vi "CompVisionUtil_ObjectToRobotPose.vi"(9 "RobotToCamera":T1={"TRANSLATION3D"={"X"=0.0, "Y"=0.0, "Z"=0.0}, "ROTATION3D"={"Q_quaternion"={"R"=1.0, "V"=[0.0, 0.0, 0.0]}}, "XF"=FALSE} {"TRANSLATION3D"."Z" format="%14.3f"; "TRANSLATION3D"."Y" format="%14.3f"; "TRANSLATION3D"."X" format="%14.3f"}, 10 "CameraToObject":T1={"TRANSLATION3D"={"X"=0.0, "Y"=0.0, "Z"=0.0}, "ROTATION3D"={"Q_quaternion"={"R"=1.0, "V"=[0.0, 0.0, 0.0]}}, "XF"=FALSE} {"TRANSLATION3D"."Z" format="%14.3f"; "TRANSLATION3D"."Y" format="%14.3f"; "TRANSLATION3D"."X" format="%14.3f"}, 11 "ObjectInField":T5={"Translation3d"={"X"=0.0, "Y"=0.0, "Z"=0.0}, "Rotation3d"={"Q_quaternion"={"R"=1.0, "V"=[0.0, 0.0, 0.0]}}} {"Translation3d"."Z" format="%14.3f"; "Translation3d"."Y" format="%14.3f"; "Translation3d"."X" format="%14.3f"}) -> (3 "ObjectToRobotPose":T5={"Translation3d"={"X"=0.0, "Y"=0.0, "Z"=0.0}, "Rotation3d"={"Q_quaternion"={"R"=1.0, "V"=[0.0, 0.0, 0.0]}}} {"Translation3d"."Z" format="%14.3f"; "Translation3d"."Y" format="%14.3f"; "Translation3d"."X" format="%14.3f"})   [LabVIEW 2019, in "Trajectory_Library.lvlib"]
doc: "Returns the robot's pose in the field coordinate system given an object's field-relative pose, the transformation from the camera's pose to the object's pose (obtained via computer vision), and the transformation from the robot's pose to the camera's pose.\n\nThe object could be a target or a fiducial marker.\n \nInputs:\n -- ObjectInField -- Pose3d -- An object's field-relative pose.\n -- CameraToObject -- Transform3d -- The transformation from the camera's pose to the object's pose. This comes from computer vision.\n -- RobotToCamera -- Transform3d -- The transformation from the robot's pose to the camera's pose. This can either be a constant for a rigidly mounted camera, or variable if the camera is mounted to\n a turret. If the camera was mounted 3 inches in front of the \"origin\" (usually physical center) of the robot, this would be new Transform3d(Units.inchesToMeters(3.0), 0.0, 0.0,\n new Rotation3d()).\n\nReturns:\n -- ObjectToRobotPose -- Pose3d -- The robot's field-relative pose."
uses:
  Trajectory_Library.lvlib
  TypeDef/TRANSLATION3D.ctl
  TypeDef/QUATERNION.ctl
  TypeDef/ROTATION3D.ctl
  TypeDef/POSE3D.ctl
  TypeDef/TRANSFORM3D.ctl
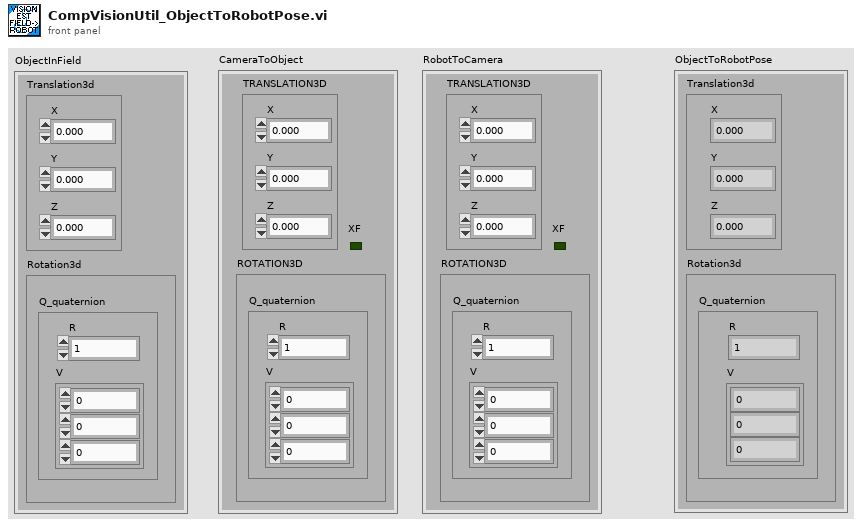
[diagram p1: front panel]
types:
  T1 = typedef "Trajectory_Library.lvlib/TRANSFORM3D.ctl" = cluster{"TRANSLATION3D":T2, "ROTATION3D":T3, "XF":bool}
  T2 = typedef "Trajectory_Library.lvlib/TRANSLATION3D.ctl" = cluster{"X":dbl, "Y":dbl, "Z":dbl}
  T3 = typedef "Trajectory_Library.lvlib/ROTATION3D.ctl" = cluster{"Q_quaternion":T4}
  T4 = typedef "Trajectory_Library.lvlib/QUATERNION.ctl" = cluster{"R":dbl, "V":dbl[]}
  T5 = typedef "Trajectory_Library.lvlib/POSE3D.ctl" = cluster{"Translation3d":T2, "Rotation3d":T3}
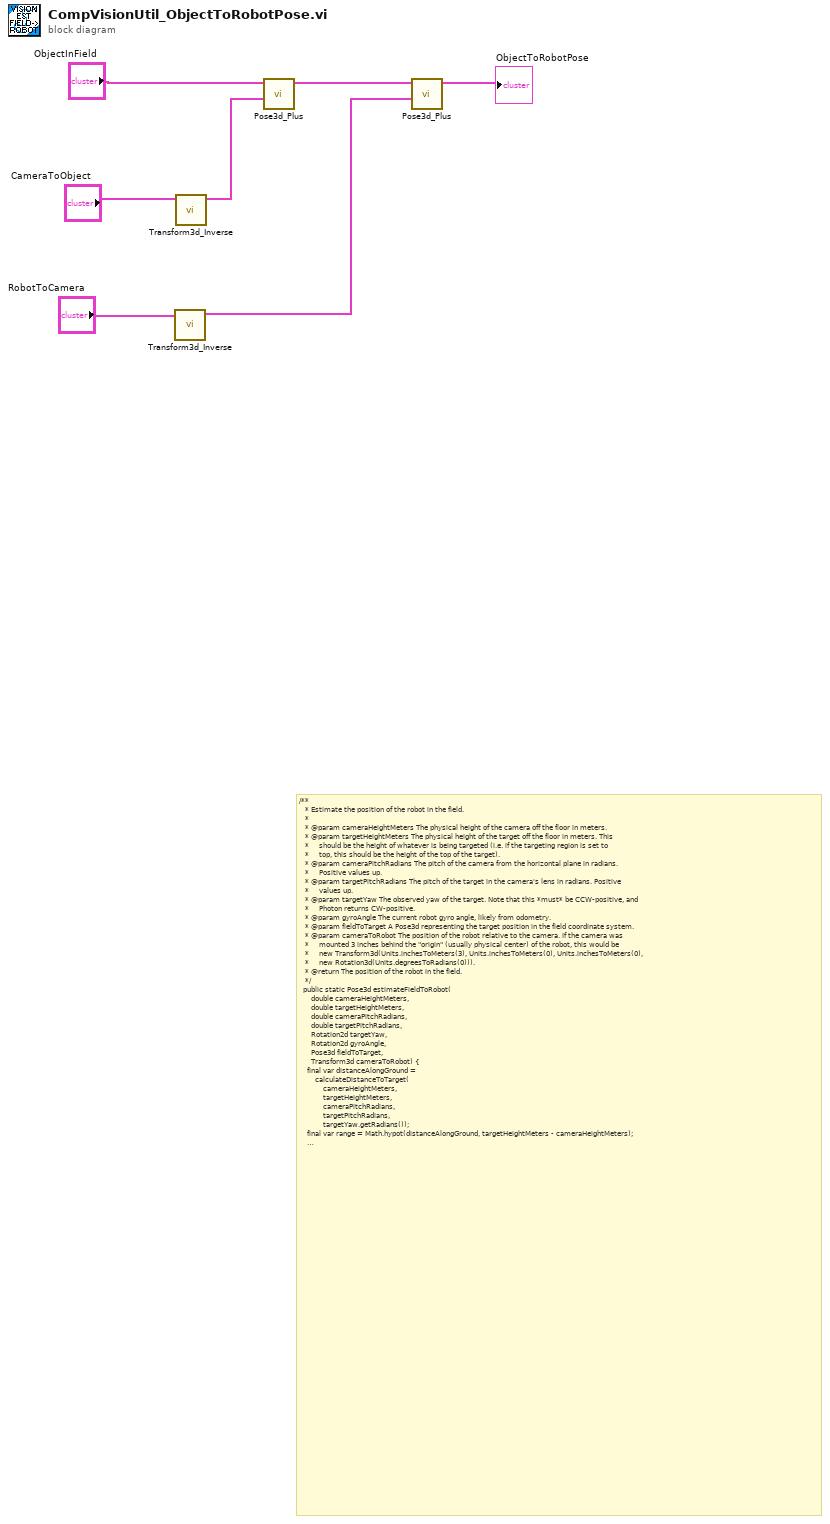
[diagram p0: block diagram]
diagram:
  # "/**\n   * Estimate the position of the robot in the field.\n   *\n   * @param cameraHeightMeters The physical height of the camera off the floor in meters.\n   * @param targetHeightMeters The physical height of the target off the floor in meters. This\n   *     should be the height of whatever is being targeted (i.e. if the targeting region is set to\n   *     top, this should be the height of the top of the target).\n   * @param cameraPitchRadians The pitch of the camera from the horizontal plane in radians.\n   *     Positive values up.\n   * @param targetPitchRadians The pitch of the target in the camera's lens in radians. Positive\n   *     values up.\n   * @param targetYaw The observed yaw of the target. Note that this *must* be CCW-positive, and\n   *     Photon returns CW-positive.\n   * @param gyroAngle The current robot gyro angle, likely from odometry.\n   * @param fieldToTarget A Pose3d representing the target position in the field coordinate system.\n   * @param cameraToRobot The position of the robot relative to the camera. If the camera was\n   *     mounted 3 inches behind the \"origin\" (usually physical center) of the robot, this would be\n   *     new Transform3d(Units.inchesToMeters(3), Units.inchesToMeters(0), Units.inchesToMeters(0),\n   *     new Rotation3d(Units.degreesToRadians(0))).\n   * @return The position of the robot in the field.\n   */\n  public static Pose3d estimateFieldToRobot(\n      double cameraHeightMeters,\n      double targetHeightMeters,\n      double cameraPitchRadians,\n      double targetPitchRadians,\n      Rotation2d targetYaw,\n      Rotation2d gyroAngle,\n      Pose3d fieldToTarget,\n      Transform3d cameraToRobot) {\n    final var distanceAlongGround =\n        calculateDistanceToTarget(\n            cameraHeightMeters,\n            targetHeightMeters,\n            cameraPitchRadians,\n            targetPitchRadians,\n            targetYaw.getRadians());\n    final var range = Math.hypot(distanceAlongGround, targetHeightMeters - cameraHeightMeters);\n    return estimateFieldToRobot(\n        estimateCameraToTarget(\n            new Translation3d(\n                range, new Rotation3d(0.0, targetPitchRadians, targetYaw.getRadians())),\n            fieldToTarget,\n            gyroAngle),\n        fieldToTarget,\n        cameraToRobot);\n  }"
  n1 = call "Transform3d_Inverse.vi"("inTransform3d"="RobotToCamera") -> ("outTransform3d"=w2:T1)  [unwired: 10 in]
  n2 = call "Transform3d_Inverse.vi"("inTransform3d"="CameraToObject") -> ("outTransform3d"=w5:T1)  [unwired: 10 in]
  n3 = call "Pose3d_Plus.vi"("other Transform3d"=w5, "in Pose3d"="ObjectInField") -> ("out Pose3d"=w4:T5)  [unwired: 9 in]
  n4 = call "Pose3d_Plus.vi"("other Transform3d"=w2, "in Pose3d"=w4) -> ("out Pose3d"=→"ObjectToRobotPose":T5)  [unwired: 9 in]
